vi "Pattern_Gen_Opcode - ChipID.vi"() -> ()   [LabVIEW 2016]
uses:
  Classes/Config_Read/Config_Read_BML.lvclass
  Classes/BML_DigiPattern_Generator/DigiPattern_Generator.lvclass
  Classes/BML_Frame_Write_Opcode/BML_Frame_Write_Opcode.lvclass
  C:/Users/8135/Desktop/BML_Pattern_Gen/BeamLink_Pattern_Gen/BML_Pattern_Gen_Refactor/Classes/BML_Frame_Root/BML_Frame_Root.lvclass
  Classes/BML_Frame_RW/BML_Frame_RW.lvclass
  Classes/BML_Frame_Read/BML_Frame_Read.lvclass
  Classes/BML_Frame_SetID/BML_Frame_SetID.lvclass
  Classes/Config_Read/RW_Option.ctl
  Classes/Config_Read/BurstLength.ctl
  Classes/Config_Read/OperationMode.ctl
  Classes/Config_Read/Frame_Data.ctl
panel:
  in  "Folder mode?":bool
  in  "Config File Path":path
  in  "Config Folder Path":path
  in  "num of wait cycle of read":i8=2
  in  "Timeset between frms":u32=40
  out "error out":errorcluster
  in  "PinMap":path
  in  "error in (no error)":errorcluster
  # "Version 1.3.2\nAdd support for chipID settings in CSV\n\nConfig folder mode"
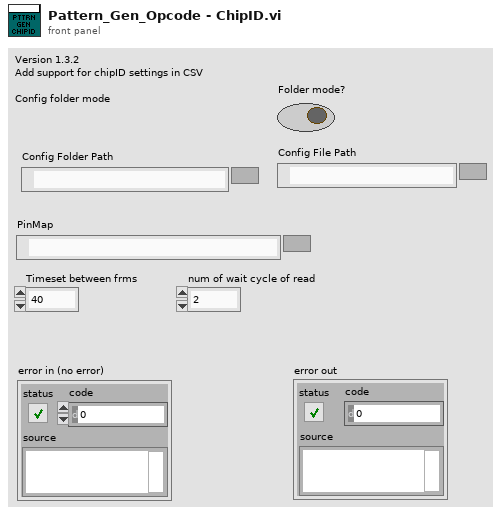
[diagram p1: front panel]
types:
  T1 = typedef "Config_Read_BML.lvclass/Frame_Data.ctl" = cluster{"Pattern_Name":string, "Operation Mode":T2, "BurstLength":T3, "FSN":u8, "Start_Addr":u16, "Data":u8[], "R/W?":T4, "Opcode":string[], "ChipID":u8, "num of wait cycle of read":i8}
  T2 = typedef "Config_Read_BML.lvclass/OperationMode.ctl" = enum8{"Normal", "ImmeEffect", "InitSlaveID", "LoadData"}
  T3 = typedef "Config_Read_BML.lvclass/BurstLength.ctl" = enum8{"0", "2", "3", "4", "5", "8", "16", "32"}
  T4 = typedef "Config_Read_BML.lvclass/RW_Option.ctl" = enum16{"Read", "Write", "R/W"}
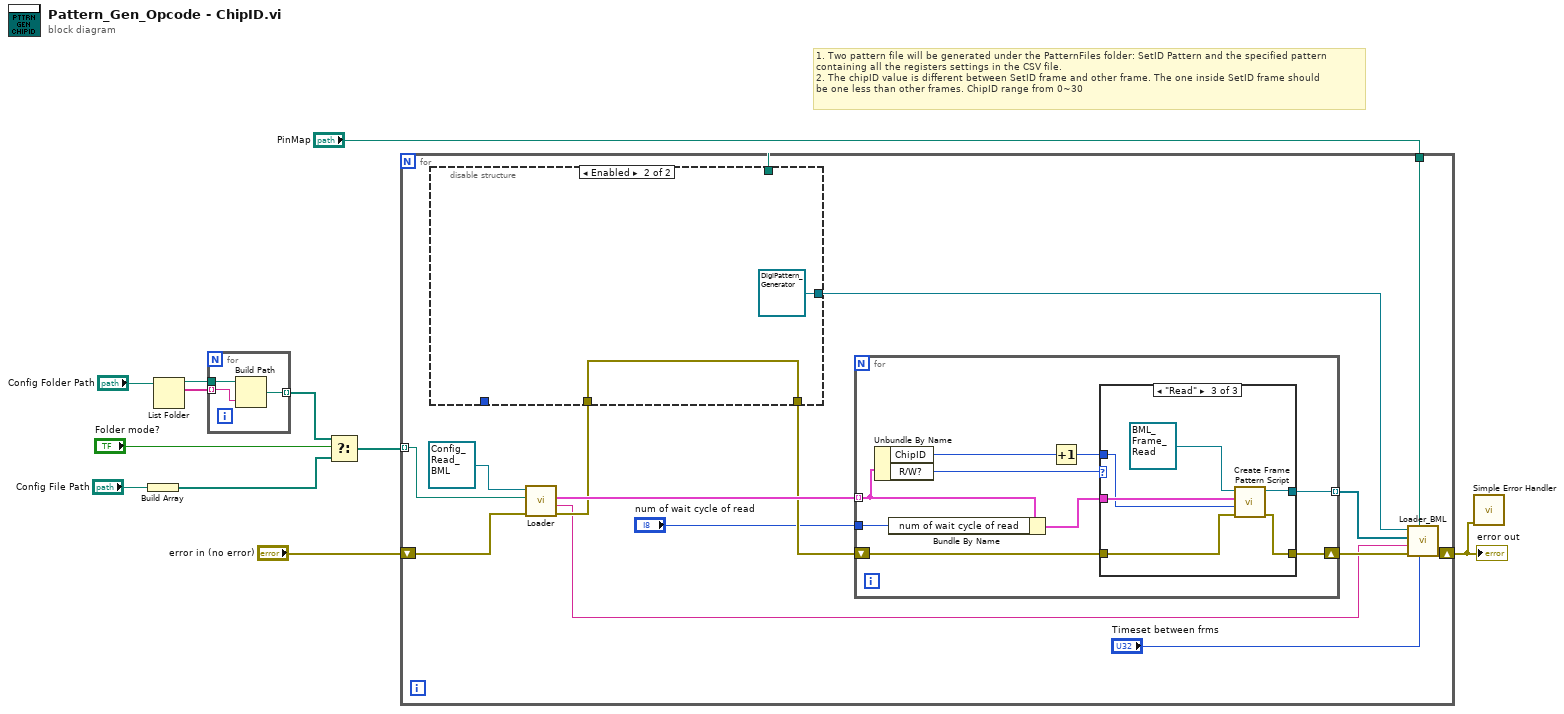
[diagram p0: block diagram]
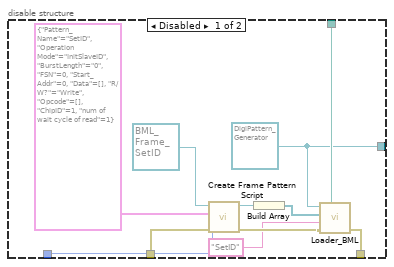
[diagram p2: hidden frame]
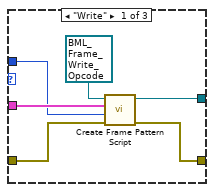
[diagram p3: hidden frame]
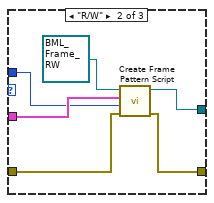
[diagram p4: hidden frame]
diagram:
  # "1. Two pattern file will be generated under the PatternFiles folder: SetID Pattern and the specified pattern\ncontaining all the registers settings in the CSV file.\n2. The chipID value is different between SetID frame and other frame. The one inside SetID frame should \nbe one less than other frames. ChipID range from 0~30"
  n1 = Build Array("Config File Path") -> (w3:path[])
  n2 = List Folder(path="Config Folder Path") -> (path out=w6:path, filenames=w7:string[])  [unwired: 3 in, 2 out]
  n3 = for {
    tunnel: w7 -> [w13] mode=indexing
    tunnel: w6 -> [w14]
    tunnel: [w12] -> w4 mode=indexing
    n4 = Build Path(base path=w14, name or relative path=w13) -> (appended path=w12:path)
  }
  n5 = Select(t=w4, s="Folder mode?", f=w3) -> (s? t:f=w1:path[])
  n6 = for {
    tunnel: "PinMap" -> [w21]
    shift-right: [w18] -> w9
    shift-left: "error in (no error)" -> [w27]
    tunnel: w1 -> [w15] mode=indexing
    n7 = call "Loader.vi"("error in (no error)"=w27, "Path"=w15, "Config_Read.lvclass"=refnum<class "Config_Read_BML.lvclass"> refnum) -> ("error out"=w25:errorcluster, "Pattern_Name"=w20:string, "FRM_Data_Array"=w26:T1[])  [unwired: 5 in, 1 out]
    n8 = disable-structure shown="Enabled" {
      disable-tunnel: w25 -> [w37 w40]
      disable-tunnel: [w36 w40] -> w24
      disable-tunnel: _ -> [w33 _]
      disable-tunnel: w21 -> [w30 _]
      disable-tunnel: [w29 refnum<class "DigiPattern_Generator.lvclass"> refnum ("BML_DigiPattern_Generator.lvclass")] -> w19
      frame Disabled {
        w29 = refnum<class "DigiPattern_Generator.lvclass"> refnum ("BML_DigiPattern_Generator.lvclass")
        n9 = call-dynamic "Create Frame Pattern Script.vi"("error in (no error)"=w37, "ChipID"=w33, "Frame_Data"=T1 {"Pattern_Name"="SetID", "Operation Mode"=enum."InitSlaveID", "BurstLength"=enum."0", "FSN"=0, "Start_Addr"=0, "Data"=[], "R/W?"=enum."Write", "Opcode"=[], "ChipID"=1, "num of wait cycle of read"=1}, "BML_Frame_SetID in"=refnum<class "BML_Frame_SetID.lvclass"> refnum ("BML_Frame_SetID.lvclass")) -> ("error out"=w35:errorcluster, "BML_Frame_SetID out"=w32:refnum<class "BML_Frame_SetID.lvclass">)  [unwired: 6 in]
        n10 = Build Array(w32) -> (w31:refnum<class "BML_Frame_SetID.lvclass">[])
        n11 = call "Loader_BML.vi"("PinMap"=w30, "error in (no error)"=w35, "Pattern Name"="SetID", "BML Frame Array"=w31, "BML_DigiPattern_Generator.lvclass"=w29) -> ("error out"=w36:errorcluster)  [unwired: 5 in, 1 out]
      }
      frame Enabled {
      }
    }
    n12 = for {
      tunnel: w26 -> [w44] mode=indexing
      shift-right: [w48] -> w23
      shift-left: w24 -> [w49]
      tunnel: [w47] -> w22 mode=indexing
      tunnel: "num of wait cycle of read" -> [w43]
      n13 = Unbundle By Name(w44) -> ("ChipID"=w46:u8, "R/W?"=w50:T4)
      n14 = Bundle By Name(cluster=w44, "num of wait cycle of read"=w43) -> (w42:T1)
      n15 = Increment(x=w46) -> (x+1=w45:u8)
      n16 = case shown="\"Read\"" w50 {
        tunnel: w49 -> [w55 w60 w66]
        tunnel: w42 -> [w56 w61 w64]
        tunnel: [w54 w58 w67] -> w47
        tunnel: [w53 w59 w65] -> w48
        tunnel: w45 -> [w51 w57 w63]
        frame "Write" {
          n17 = call-dynamic "Create Frame Pattern Script.vi"("error in (no error)"=w55, "ChipID"=w51, "Frame_Data"=w56, "BML_Frame_Write_Opcode in"=refnum<class "BML_Frame_Write_Opcode.lvclass"> refnum ("BML_Frame_Write_Opcode.lvclass")) -> ("error out"=w53:errorcluster, "BML_Frame_Write_Opcode out"=w54:refnum<class "BML_Frame_Write_Opcode.lvclass">)  [unwired: 6 in]
        }
        frame "R/W" {
          n18 = call-dynamic "Create Frame Pattern Script.vi"("error in (no error)"=w60, "ChipID"=w57, "Frame_Data"=w61, "BML_Frame_RW in"=refnum<class "BML_Frame_RW.lvclass"> refnum ("BML_Frame_RW.lvclass")) -> ("error out"=w59:errorcluster, "BML_Frame_RW out"=w58:refnum<class "BML_Frame_RW.lvclass">)  [unwired: 6 in]
        }
        frame "Read" {
          n19 = call-dynamic "Create Frame Pattern Script.vi"("error in (no error)"=w66, "ChipID"=w63, "Frame_Data"=w64, "BML_Frame_Read in"=refnum<class "BML_Frame_Read.lvclass"> refnum ("BML_Frame_Read.lvclass")) -> ("error out"=w65:errorcluster, "BML_Frame_Read out"=w67:refnum<class "BML_Frame_Read.lvclass">)  [unwired: 6 in]
        }
      }
    }
    n20 = call "Loader_BML.vi"("Timeset between frms"="Timeset between frms", "PinMap"=w21, "error in (no error)"=w23, "Pattern Name"=w20, "BML Frame Array"=w22, "BML_DigiPattern_Generator.lvclass"=w19) -> ("error out"=w18:errorcluster)  [unwired: 4 in, 1 out]
  }
  "error out" <- w9
  n21 = call <vilib>:"Simple Error Handler.vi"("error in (no error)"=w9) -> ()  [unwired: 4 in, 5 out]
